vi "Compte-resultat.vi"(1 "Argent ventes":dbl, 2 "Impots":dbl) -> (0 "Compte résultat":dbl)   [LabVIEW 2024]
uses:
  charge_salairial.vi
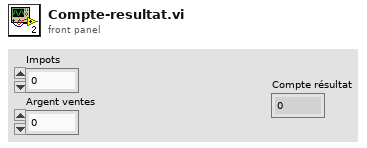
[diagram p1: front panel]
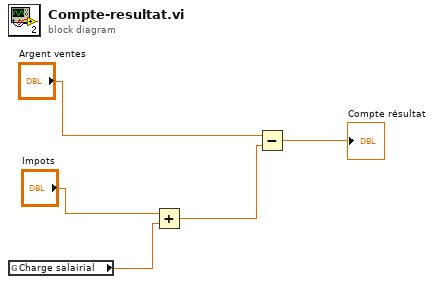
[diagram p0: block diagram]
diagram:
  n1 = global read "charge_salairial.vi" "Charge salairial"() -> (w3:dbl)
  n2 = Add(x="Impots", y=w3) -> (x+y=w2:dbl)
  n3 = Subtract(x="Argent ventes", y=w2) -> (x-y=→"Compte résultat":dbl)
